vi "Building_Alignment.vi"() -> ()   [LabVIEW 2010]
uses:
  Anemometry Sub Vis/Controls/User_Specific_mode.ctl
  Anemometry Sub Vis/Controls/Tunnel_Coordinates.ctl
  Anemometry Sub Vis/Gen Trav/Trav_mode.ctl
  Anemometry Sub Vis/Globals/Trav_pos_global.vi
  Anemometry Sub Vis/Globals/Meas_global.vi
  Anemometry Sub Vis/Globals/Preference_global.vi
  Anemometry Sub Vis/Gen Trav/Route mapping/Route_mapping_global.vi
panel:
  out "Building Names":string[](array[string])
  out "Corners":dbl[][][](array[numeric])
  in  "Vertical Height":dbl=500.0
  in  "Selected Buildings":i32[](listbox)
  in  "Mode":T1(ring)
  out "Original Position":dbl[](array[numeric]) format="%.2f"
  in  "Traverse Position":dbl[](array[numeric])=[0.0, 0.0, 0.0] format="%.2f"
  out "Message":string
  in  "Go Back":bool
  in  "OK":bool
  in  "stop":bool
  # "X                 Y              Z"
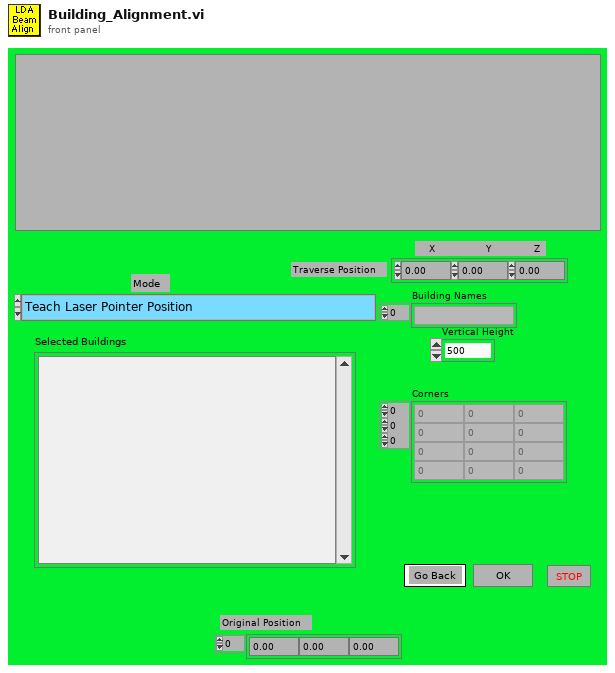
[diagram p1: front panel]
types:
  T1 = enum16{"Teach Laser Pointer Position", "Visit Corners of Selected buidings"}
  T2 = typedef "User_Specific_mode.ctl" = enum16{"Check VI only", "Run VI"}
  T3 = typedef "Tunnel_Coordinates.ctl" = enum16{"Work in Tunnel Coordinates", "Work in Model Coordinates"}
  T4 = typedef "Trav_mode.ctl" = enum16{"Move traverse", "Read traverse position", "Teach Position"}
  T5 = enum16{"Load From Excel File", "Save to Excel File"}
  T6 = enum16{"To Traverse Coordinates", "To User Coordinates"}
  T7 = typedef "Exclude_cluster.ctl" = cluster{"Sizes":T8, "Name":string, "Exclude Type":T9}
  T8 = typedef "Box_size.ctl" = cluster{"Max":dbl, "Min":dbl}[]
  T9 = typedef "Exclusion_type.ctl" = enum16{"Exclude completely", "Allow only vertical moves"}
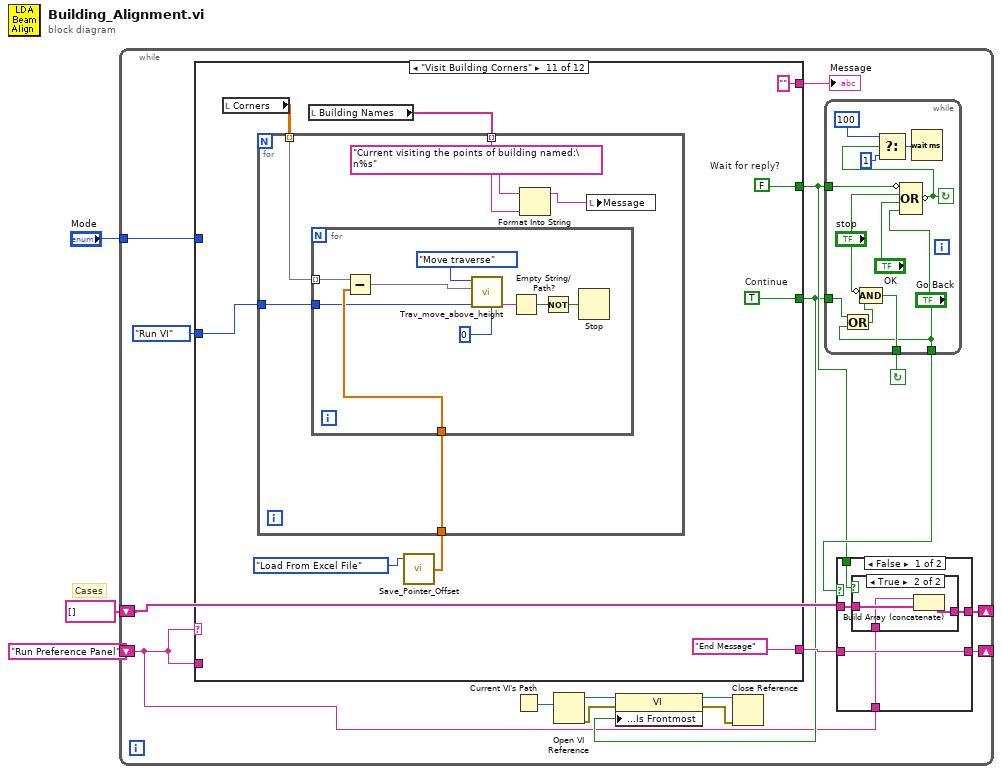
[diagram p0: block diagram]
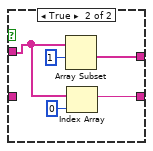
[diagram p3: hidden frame]
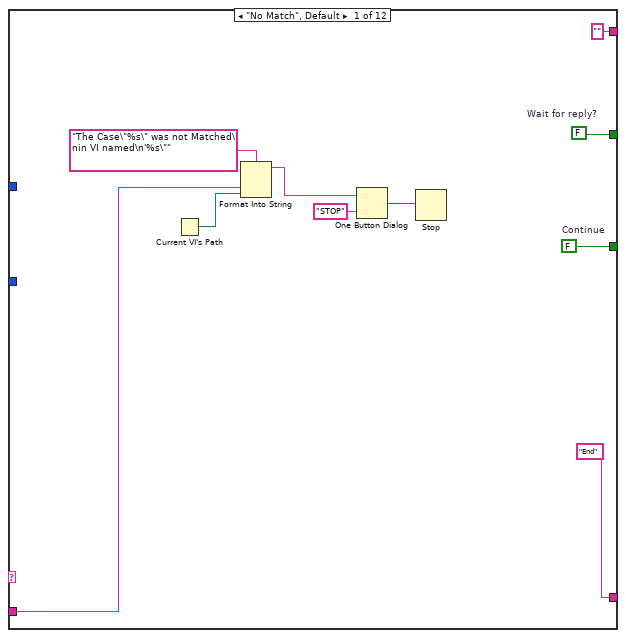
[diagram p4: hidden frame]
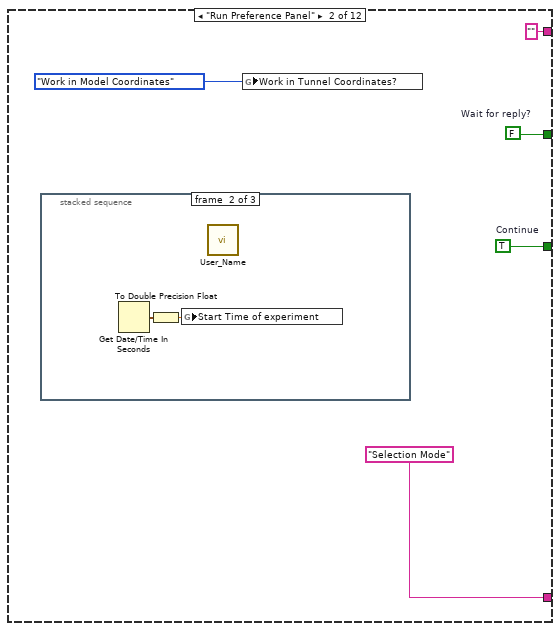
[diagram p5: hidden frame]
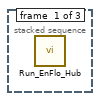
[diagram p6: hidden frame]
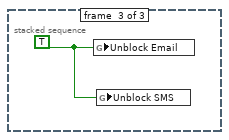
[diagram p7: hidden frame]
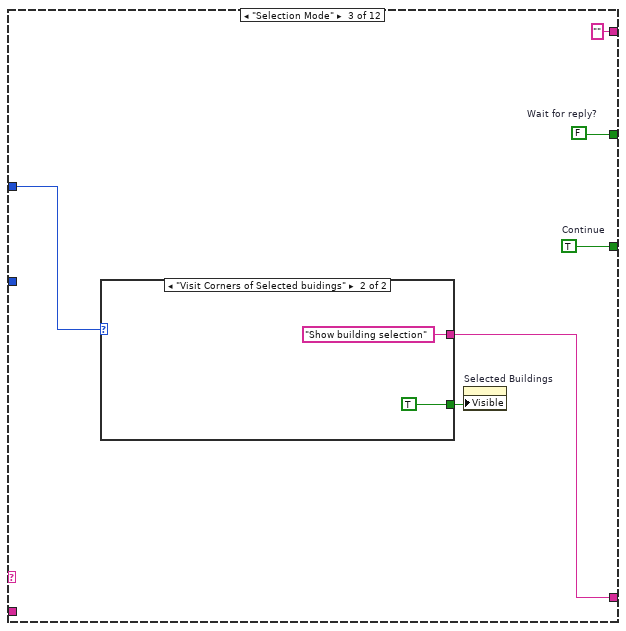
[diagram p8: hidden frame]
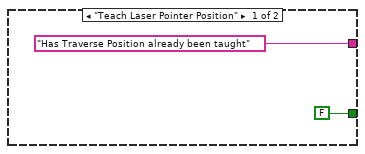
[diagram p9: hidden frame]
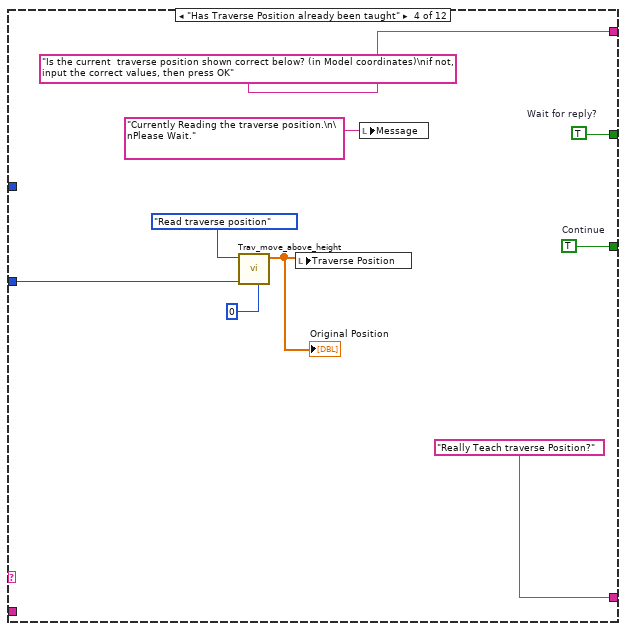
[diagram p10: hidden frame]
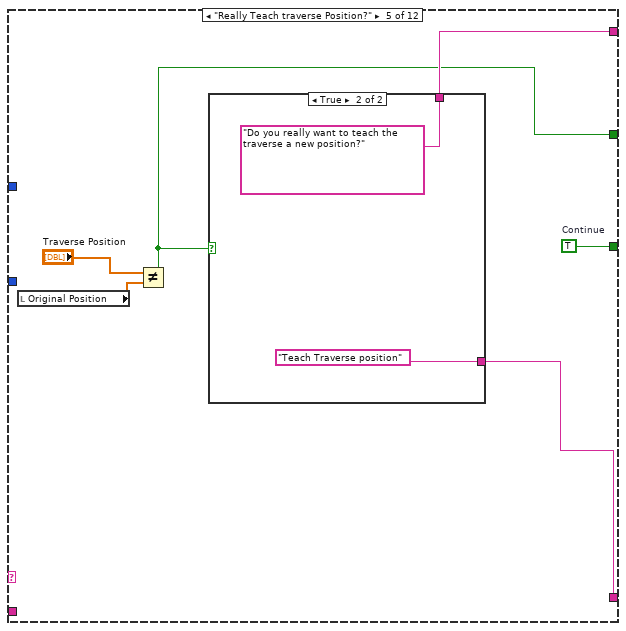
[diagram p11: hidden frame]
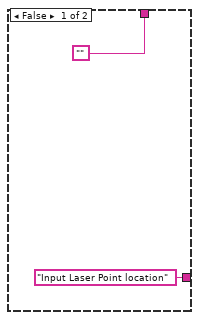
[diagram p12: hidden frame]
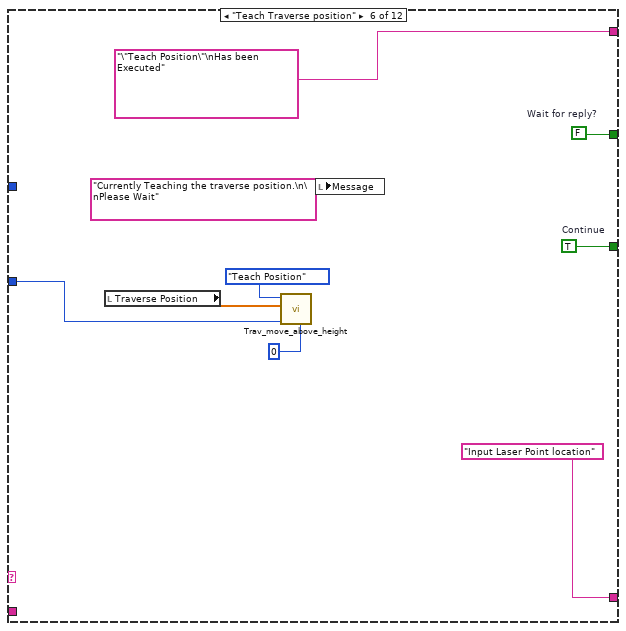
[diagram p13: hidden frame]
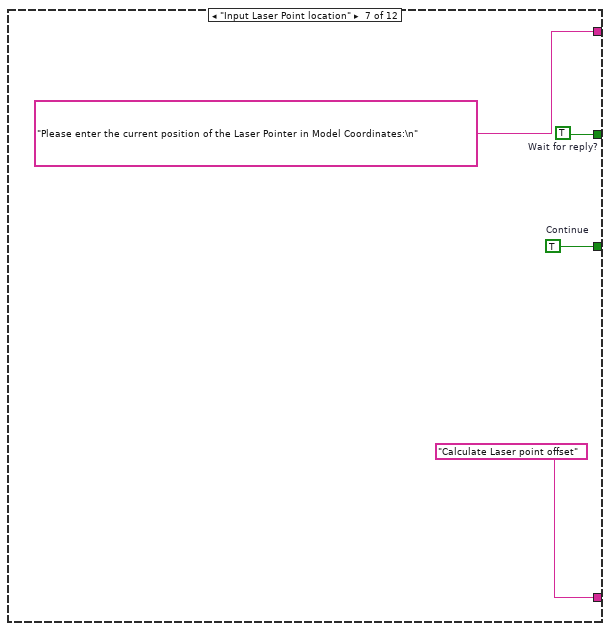
[diagram p14: hidden frame]
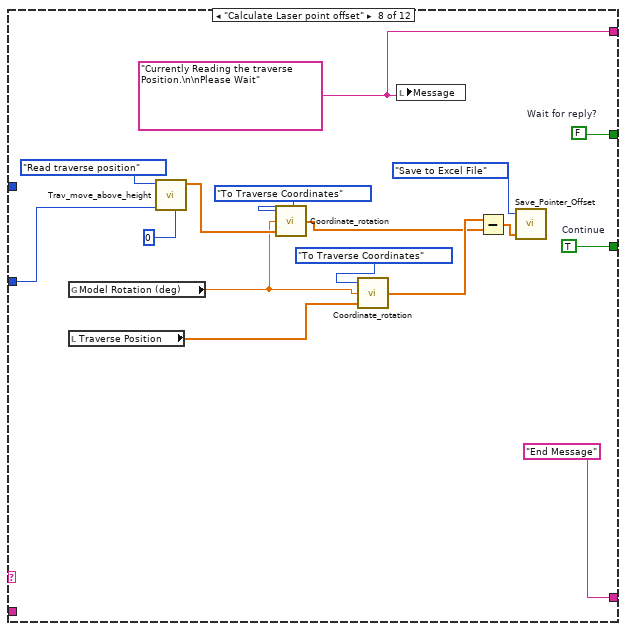
[diagram p15: hidden frame]
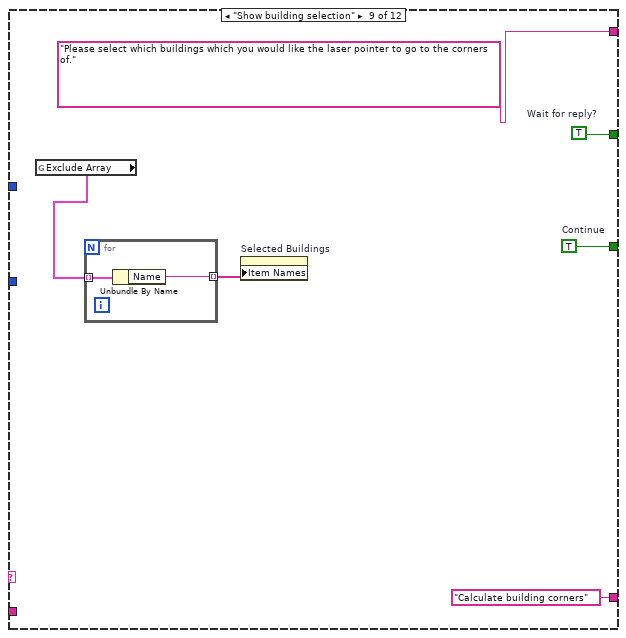
[diagram p16: hidden frame]
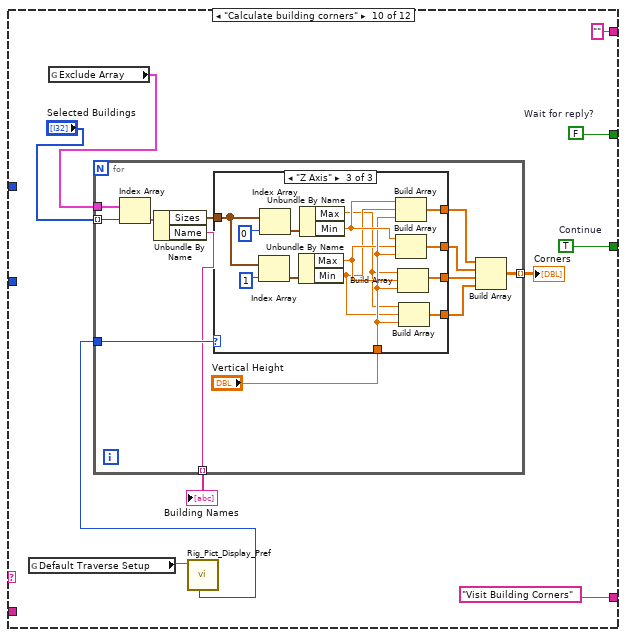
[diagram p17: hidden frame]
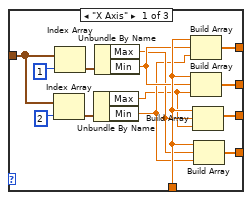
[diagram p18: hidden frame]
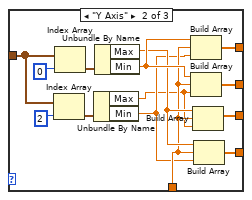
[diagram p19: hidden frame]
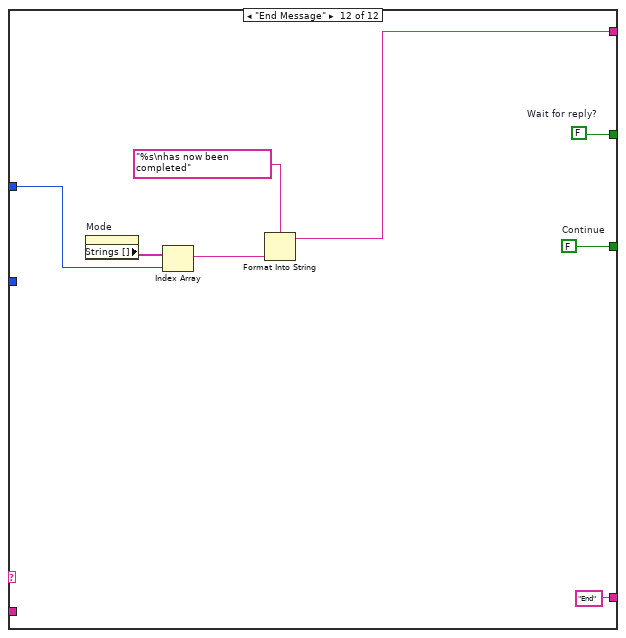
[diagram p20: hidden frame]
diagram:
  # "Cases"
  n1 = while {
    tunnel: "Mode" -> [w5]
    shift-left: string[] [] -> [w18]
    shift-right: [w17] -> _
    shift-left: "Run Preference Panel" -> [w4]
    shift-right: [w16] -> _
    stop <- w20 continue-if-true
    n2 = case shown="\"Visit Building Corners\"" w4 {
      tunnel: [w55 w60 w69 w82 w88 w101 w105 w121 w127 w137 w200 w225] -> w6
      tunnel: ["End" "Selection Mode" w65 "Really Teach traverse Position?" w83 "Input Laser Point location" "Calculate Laser point offset" "End Message" "Calculate building corners" "Visit Building Corners" "End Message" "End"] -> w15
      tunnel: [w54 w59 w68 w81 w84 w100 w104 w120 w126 w138 w201 w224] -> w7
      tunnel: ["" "" "" "Is the current  traverse position shown correct below? (in Model coordinates)\nif not, input the correct values, then press OK" w87 "\"Teach Position\"\nHas been Executed" "Please enter the current position of the Laser Pointer in Model Coordinates:\n" w116 "Please select which buildings which you would like the laser pointer to go to the corners of." "" "" w218] -> w14
      tunnel: User_Specific_mode."Run VI" ("Simulate/Run") -> [_ _ _ w77 _ w96 _ w117 _ _ w195 _]
      tunnel: w5 -> [_ _ w66 _ _ _ _ _ _ _ _ w221]
      tunnel: w4 -> [w46 _ _ _ _ _ _ _ _ _ _ _]
      frame "No Match", Default {
        w54 = FALSE  # Wait for reply?
        w55 = FALSE  # Continue
        n3 = Current VI's Path() -> (path=w47:path)
        n4 = Format Into String(format string="The Case\"%s\" was not Matched\nin VI named\n'%s\"" ("Format String"), w46, w47) -> (resulting string=w50:string)  [unwired: 2 in, 1 out]
        n5 = One Button Dialog(message=w50, button name ("OK")="STOP") -> (true=w48:bool)
        n6 = Stop(stop? (T)=w48) -> ()
      }
      frame "Run Preference Panel" {
        w59 = FALSE  # Wait for reply?
        w60 = TRUE  # Continue
        n7 = stacked-sequence {
          frame #0 {
            n8 = call "Run_EnFlo_Hub.vi"() -> ()  [unwired: 8 in]
          }
          frame #1 {
            n9 = Get Date/Time In Seconds() -> (seconds since 1Jan1904=w62:timestamp)
            n10 = To Double Precision Float(number=w62) -> (double precision float=w61:dbl)
            n11 = global write "Meas_global.vi" "Start Time of experiment"(w61) -> ()
            n12 = call "User_Name.vi"() -> ()  [unwired: 1 out]
          }
          frame #2 {
            w63 = TRUE
            n13 = global write "Preference_global.vi" "Unblock Email"(w63) -> ()
            n14 = global write "Preference_global.vi" "Unblock SMS"(w63) -> ()
          }
        }
        n15 = global write "Trav_pos_global.vi" "Work in Tunnel Coordinates?"(Tunnel_Coordinates."Work in Model Coordinates" ("Work in Tunnel Coordinates?")) -> ()
      }
      frame "Selection Mode" {
        w68 = FALSE  # Wait for reply?
        w69 = TRUE  # Continue
        n16 = case shown="\"Visit Corners of Selected buidings\"" w66 {
          tunnel: ["Has Traverse Position already been taught" "Show building selection"] -> w65
          tunnel: [FALSE TRUE] -> w64
          frame "Teach Laser Pointer Position" {
          }
          frame "Visit Corners of Selected buidings" {
          }
        }
        n17 = property on="Selected Buildings" class="LstBox (strict)"("Visible"=w64) -> ()  [unwired: 2 in, 2 out]
      }
      frame "Has Traverse Position already been taught" {
        w81 = TRUE  # Wait for reply?
        w82 = TRUE  # Continue
        n18 = call "Trav_move_above_height.vi"("Currently on Point"=0, "Simulate/Run"=w77, "Mode"=Trav_mode."Read traverse position") -> ("Trav Position achieved"=w76:dbl[])  [unwired: 7 in, 1 out]
        "Original Position" <- w76
        n19 = local write "Traverse Position"(w76) -> ()
        n20 = local write "Message"("Currently Reading the traverse position.\n\nPlease Wait." ("Message")) -> ()
      }
      frame "Really Teach traverse Position?" {
        w88 = TRUE  # Continue
        n21 = local read "Original Position"() -> (w86:dbl[])
        n22 = Not Equal?(x="Traverse Position", y=w86) -> (x != y?=w84:bool)
        n23 = case shown="True" w84 {
          tunnel: ["" "Do you really want to teach the traverse a new position?"] -> w87
          tunnel: ["Input Laser Point location" "Teach Traverse position"] -> w83
          frame False {
          }
          frame True {
          }
        }
      }
      frame "Teach Traverse position" {
        w100 = FALSE  # Wait for reply?
        w101 = TRUE  # Continue
        n24 = local read "Traverse Position"() -> (w95:dbl[])
        n25 = call "Trav_move_above_height.vi"("Currently on Point"=0, "Simulate/Run"=w96, "New Position"=w95, "Mode"=Trav_mode."Teach Position") -> ()  [unwired: 6 in, 2 out]
        n26 = local write "Message"("Currently Teaching the traverse position.\n\nPlease Wait" ("Message")) -> ()
      }
      frame "Input Laser Point location" {
        w104 = TRUE  # Wait for reply?
        w105 = TRUE  # Continue
      }
      frame "Calculate Laser point offset" {
        w116 = "Currently Reading the traverse Position.\n\nPlease Wait"
        w120 = FALSE  # Wait for reply?
        w121 = TRUE  # Continue
        n27 = global read "Trav_pos_global.vi" "Model Rotation (deg)"() -> (w113:dbl)
        n28 = local read "Traverse Position"() -> (w112:dbl[])
        n29 = call "Trav_move_above_height.vi"("Currently on Point"=0, "Simulate/Run"=w117, "Mode"=Trav_mode."Read traverse position") -> ("Trav Position achieved"=w115:dbl[])  [unwired: 7 in, 1 out]
        n30 = call "Coordinate_rotation.vi"("Input Position"=w115, "Coordinate rotation (deg)"=w113, "Mode"=T6."To Traverse Coordinates") -> ("Output Position"=w109:dbl[])
        n31 = call "Coordinate_rotation.vi"("Input Position"=w112, "Coordinate rotation (deg)"=w113, "Mode"=T6."To Traverse Coordinates") -> ("Output Position"=w110:dbl[])
        n32 = local write "Message"(w116) -> ()
        n33 = Subtract(x=w110, y=w109) -> (x-y=w107:dbl[])
        n34 = call "Save_Pointer_Offset.vi"("Values"=w107, "Mode"=T5."Save to Excel File") -> ()  [unwired: 1 in, 1 out]
      }
      frame "Show building selection" {
        w126 = TRUE  # Wait for reply?
        w127 = TRUE  # Continue
        n35 = global read "Route_mapping_global.vi" "Exclude Array"() -> (w124:T7[])
        n36 = for {
          tunnel: w124 -> [w129] mode=indexing
          tunnel: [w128] -> w123 mode=indexing
          n37 = Unbundle By Name(w129) -> ("Name"=w128:string)
        }
        n38 = property on="Selected Buildings" class="LstBox (strict)"("Item Names"=w123) -> ()  [unwired: 2 in, 2 out]
      }
      frame "Calculate building corners" {
        w138 = FALSE  # Wait for reply?
        w137 = TRUE  # Continue
        n39 = global read "Trav_pos_global.vi" "Default Traverse Setup"() -> (w133:string)
        n40 = global read "Route_mapping_global.vi" "Exclude Array"() -> (w135:T7[])
        n41 = call "Rig_Pict_Display_Pref.vi"("Traverse Name"=w133) -> ("Which Axis is vertical?"=w132:enum16{"X Axis", "Y Axis", "Z Axis"})  [unwired: 3 in, 4 out]
        n42 = for {
          tunnel: w135 -> [w151]
          tunnel: "Selected Buildings" -> [w150] mode=indexing
          tunnel: w132 -> [w146]
          tunnel: [w141] -> w131 mode=indexing
          tunnel: [w140] -> w130 mode=indexing
          n43 = Index Array(array=w151, index=w150) -> (element=w149:T7)
          n44 = Unbundle By Name(w149) -> ("Sizes"=w148:T8, "Name"=w140:string)
          n45 = case shown="\"Z Axis\"" w146 {
            tunnel: w148 -> [w162 w176 w190]
            tunnel: "Vertical Height" -> [w156 w168 w187]
            tunnel: [w160 w172 w183] -> w145
            tunnel: [w159 w171 w182] -> w144
            tunnel: [w158 w170 w181] -> w143
            tunnel: [w157 w169 w180] -> w142
            frame "X Axis" {
              n46 = Index Array(array=w162, index=2) -> (element=w164:cluster{"Max":dbl, "Min":dbl})
              n47 = Index Array(array=w162, index=1) -> (element=w165:cluster{"Max":dbl, "Min":dbl})
              n48 = Unbundle By Name(w164) -> ("Max"=w152:dbl, "Min"=w153:dbl)
              n49 = Unbundle By Name(w165) -> ("Max"=w154:dbl, "Min"=w155:dbl)
              n50 = Build Array(w156, w155, w153) -> (w160:dbl[])
              n51 = Build Array(w156, w155, w152) -> (w159:dbl[])
              n52 = Build Array(w156, w154, w152) -> (w158:dbl[])
              n53 = Build Array(w156, w154, w153) -> (w157:dbl[])
            }
            frame "Y Axis" {
              n54 = Index Array(array=w176, index=2) -> (element=w178:cluster{"Max":dbl, "Min":dbl})
              n55 = Index Array(array=w176, index=0) -> (element=w179:cluster{"Max":dbl, "Min":dbl})
              n56 = Unbundle By Name(w178) -> ("Max"=w166:dbl, "Min"=w167:dbl)
              n57 = Unbundle By Name(w179) -> ("Max"=w173:dbl, "Min"=w174:dbl)
              n58 = Build Array(w174, w168, w167) -> (w172:dbl[])
              n59 = Build Array(w174, w168, w166) -> (w171:dbl[])
              n60 = Build Array(w173, w168, w166) -> (w170:dbl[])
              n61 = Build Array(w173, w168, w167) -> (w169:dbl[])
            }
            frame "Z Axis" {
              n62 = Index Array(array=w190, index=1) -> (element=w192:cluster{"Max":dbl, "Min":dbl})
              n63 = Index Array(array=w190, index=0) -> (element=w193:cluster{"Max":dbl, "Min":dbl})
              n64 = Unbundle By Name(w192) -> ("Max"=w186:dbl, "Min"=w185:dbl)
              n65 = Unbundle By Name(w193) -> ("Max"=w184:dbl, "Min"=w188:dbl)
              n66 = Build Array(w188, w185, w187) -> (w183:dbl[])
              n67 = Build Array(w188, w186, w187) -> (w182:dbl[])
              n68 = Build Array(w184, w186, w187) -> (w181:dbl[])
              n69 = Build Array(w184, w185, w187) -> (w180:dbl[])
            }
          }
          n70 = Build Array(w145, w144, w143, w142) -> (w141:dbl[][])
        }
        "Corners" <- w131
        "Building Names" <- w130
      }
      frame "Visit Building Corners" {
        w201 = FALSE  # Wait for reply?
        w200 = TRUE  # Continue
        n71 = local read "Corners"() -> (w197:dbl[][][])
        n72 = local read "Building Names"() -> (w194:string[])
        n73 = call "Save_Pointer_Offset.vi"("Mode"=T5."Load From Excel File") -> ("Values Out"=w196:dbl[])  [unwired: 2 in]
        n74 = for {
          tunnel: w197 -> [w208] mode=indexing
          tunnel: w196 -> [w207]
          tunnel: w194 -> [w206] mode=indexing
          tunnel: w195 -> [w203]
          n75 = for {
            tunnel: w208 -> [w217] mode=indexing
            tunnel: w207 -> [w216]
            tunnel: w203 -> [w212]
            n76 = Subtract(x=w217, y=w216) -> (x-y=w213:dbl[])
            n77 = call "Trav_move_above_height.vi"("Currently on Point"=0, "Simulate/Run"=w212, "New Position"=w213, "Mode"=Trav_mode."Move traverse") -> ("Error String"=w211:string)  [unwired: 6 in, 1 out]
            n78 = Empty String/Path?(string/path=w211) -> (empty?=w210:bool)
            n79 = Not(x=w210) -> (.not. x?=w209:bool)
            n80 = Stop(stop? (T)=w209) -> ()
          }
          n81 = Format Into String(format string="Current visiting the points of building named:\n%s", w206) -> (resulting string=w204:string)  [unwired: 2 in, 1 out]
          n82 = local write "Message"(w204) -> ()
        }
      }
      frame "End Message" {
        w224 = FALSE  # Wait for reply?
        w225 = FALSE  # Continue
        n83 = property on="Mode" class="Enum (strict)"() -> ("Strings []"=w222:string[])  [unwired: 2 in, 2 out]
        n84 = Index Array(array=w222, index=w221) -> (element=w220:string)
        n85 = Format Into String(format string="%s\nhas now been completed" ("Format String"), w220) -> (resulting string=w218:string)  [unwired: 2 in, 1 out]
      }
    }
    "Message" <- w14
    n86 = Current VI's Path() -> (path=w12:path)
    n87 = Open VI Reference(vi path=w12) -> (vi reference=w11:refnum<vi>, error out=w10:errorcluster)  [unwired: 5 in]
    n88 = property class="VI"(reference=w11, error in=w10, "Front Panel Window:Is Frontmost"=w6) -> (reference out=w9:refnum<vi>, error out=w8:errorcluster)
    n89 = Close Reference(reference=w9, error in (no error)=w8) -> ()  [unwired: 1 out]
    n90 = while {
      tunnel: ["Go Back"] -> w19
      tunnel: [w28] -> w20
      tunnel: w6 -> [w27]
      tunnel: w7 -> [w30]
      stop <- w24 continue-if-true
      n91 = Or(x=w27, y="Go Back") -> (x .or. y?=w25:bool)
      n92 = Compound Arithmetic op=AND(invert "stop", w25) -> (w28:bool)
      n93 = Compound Arithmetic op=OR(invert w30, "stop", "OK", "Go Back") -> (invert w24:bool)
      n94 = Select(t=u32 100 ("millisecond timer value"), s=w24, f=u32 1) -> (s? t:f=w21:u32)
      n95 = Wait (ms)(milliseconds to wait=w21) -> ()  [unwired: 1 out]
    }
    n96 = case shown="False" w19 {
      tunnel: w18 -> [w36 w41]
      tunnel: [w35 w42] -> w17
      tunnel: w4 -> [w33 _]
      tunnel: [w34 w43] -> w16
      tunnel: w15 -> [w34 _]
      tunnel: w7 -> [w32 _]
      frame False {
        n97 = case shown="True" w32 {
          tunnel: w36 -> [w37 w40]
          tunnel: [w37 w39] -> w35
          tunnel: w33 -> [_ w38]
          frame False {
          }
          frame True {
            n98 = Build Array (concatenate)(w38, w40) -> (w39:string[])
          }
        }
      }
      frame True {
        n99 = Array Subset(array=w41, index=1 ("Array Index")) -> (w42:string[])  [unwired: 1 in]
        n100 = Index Array(array=w41, index=0 ("Index")) -> (element=w43:string)
      }
    }
  }
